vi "Quizz1.vi"() -> ()   [LabVIEW 2020]
uses:
  <vilib>/regexp/Match Regular Expression.xnode
panel:
  out "appended array 2":string[][](array[string])
  out "appended array":string[](array[string])
  out "result string 3":string
  out "result string 2":string
  out "result string":string
  out "LED 3":bool
  in  "PULSADOR 3":bool
  out "LED 2":bool
  in  "PULSADOR 2":bool
  out "LED 1":bool
  in  "PULSADOR 1":bool
  out "Contador":i32
  out "offset past number":i32
  in  "Ingrese la trama":string
  out "Respuestas":string
  in  "Ingreso de comandos":string
  in  "Ingresar":bool
  # "Quiz 1"
  # "Juan Camilo Osorio Bustamante - Diego Alejandro Vallejo Pacheco"
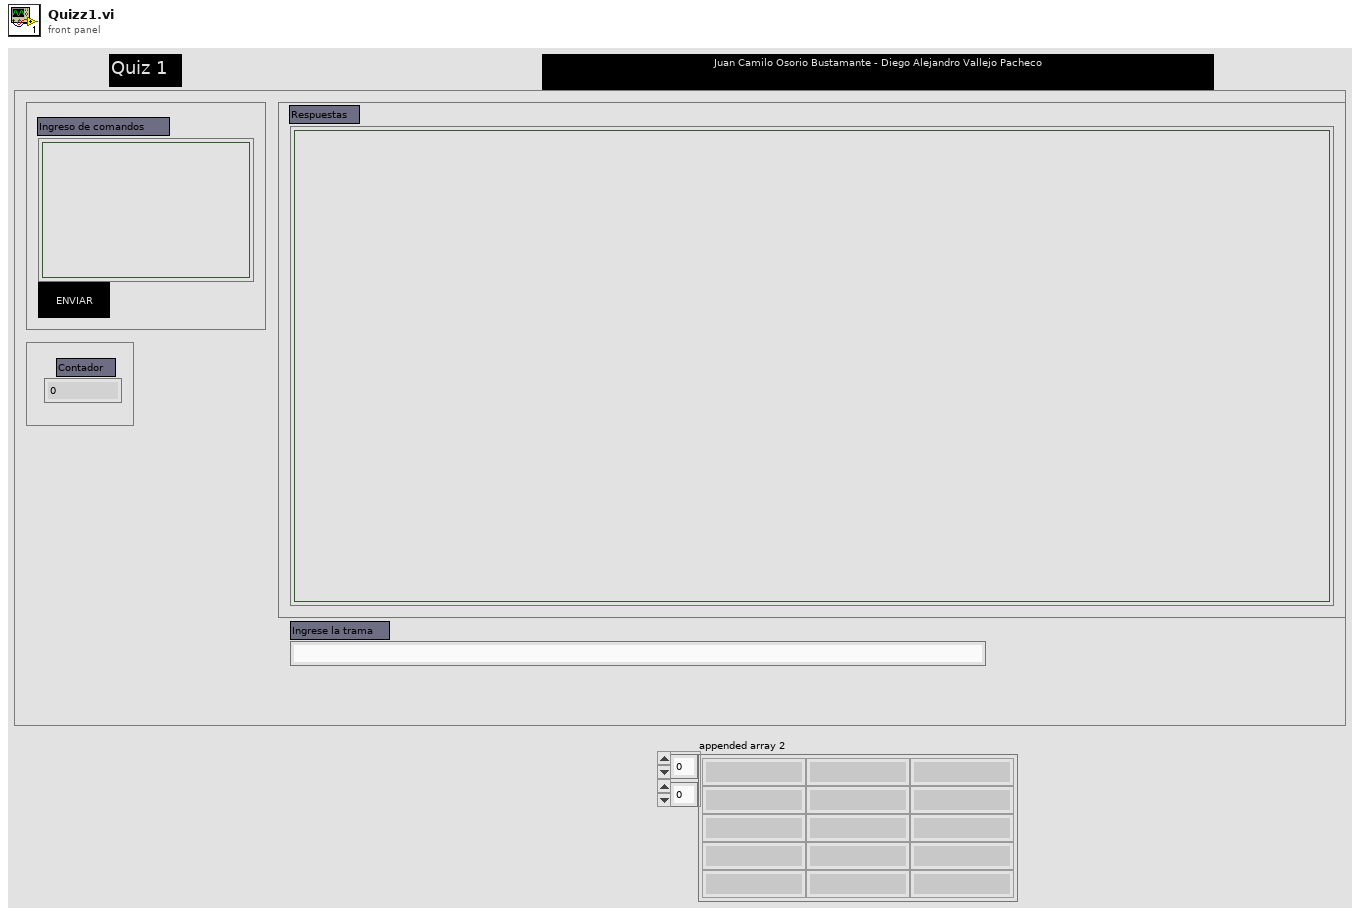
[diagram p1: front panel]
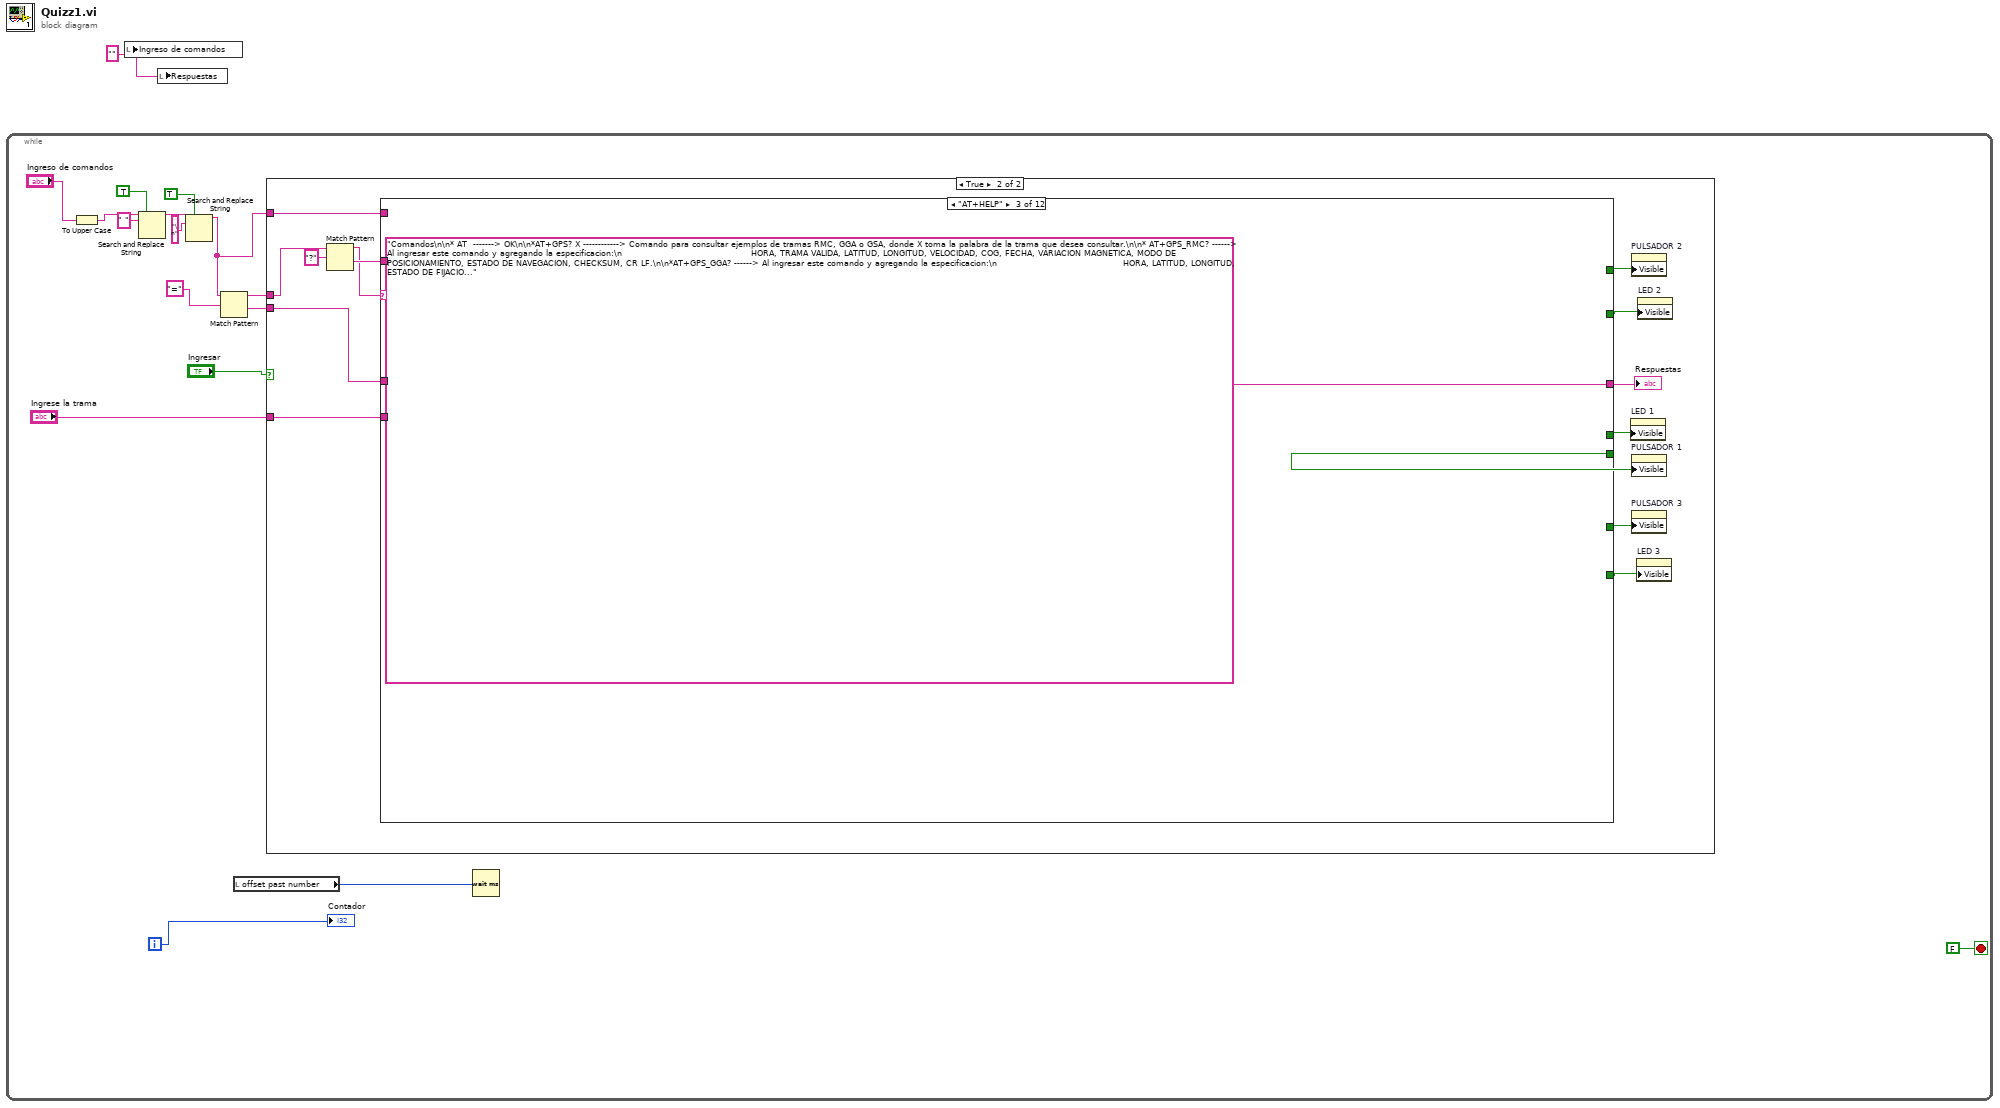
[diagram p0: block diagram]
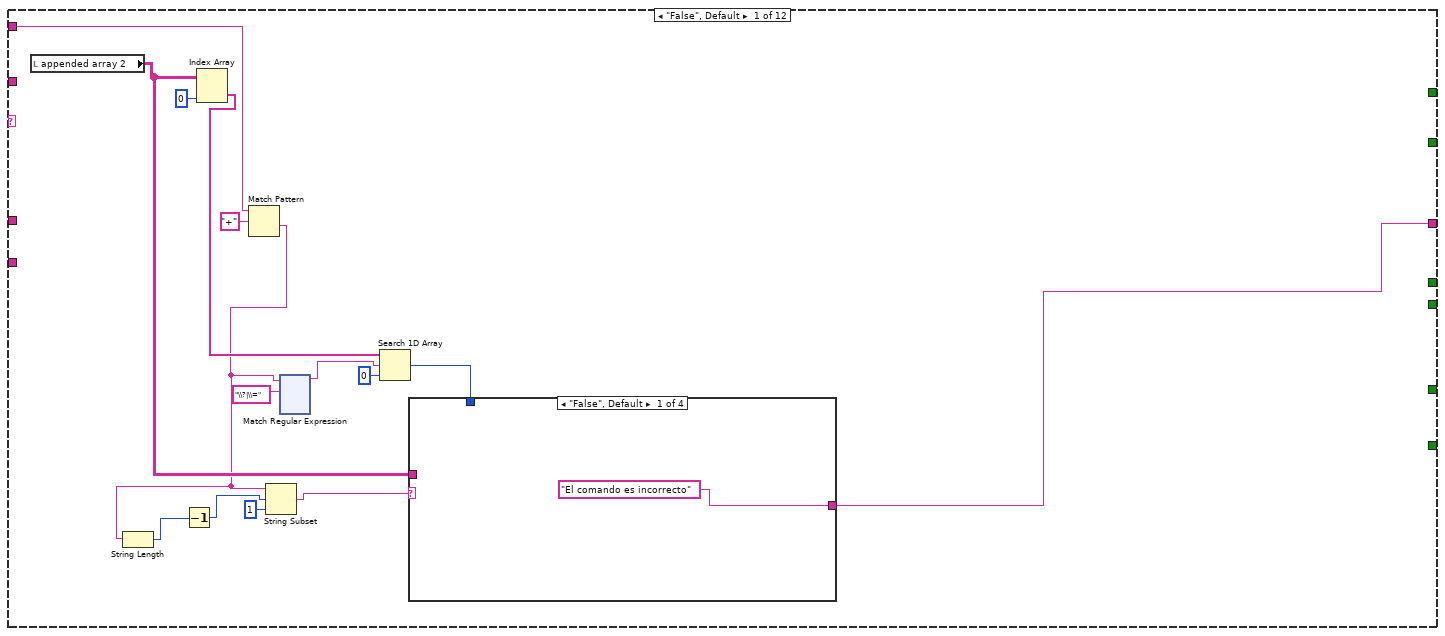
[diagram p3: hidden frame]
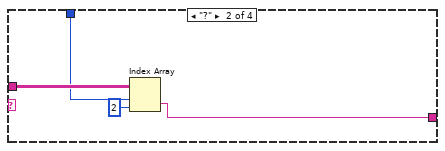
[diagram p4: hidden frame]
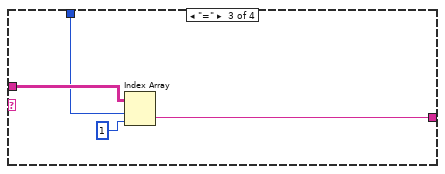
[diagram p5: hidden frame]
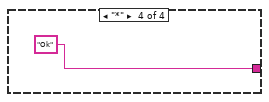
[diagram p6: hidden frame]
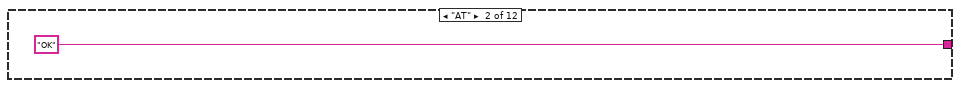
[diagram p7: hidden frame]
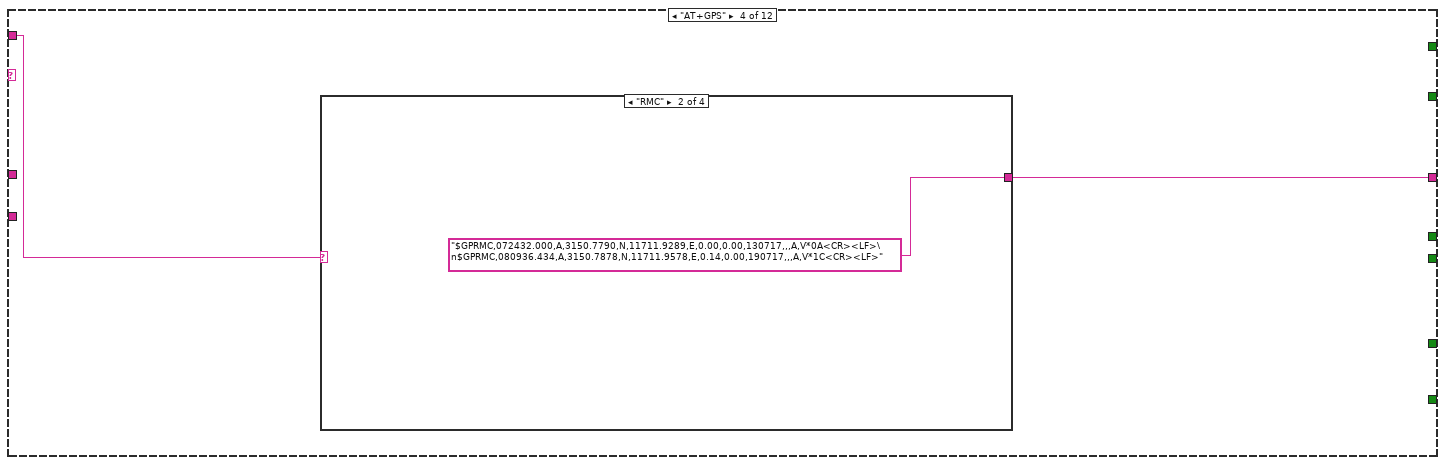
[diagram p8: hidden frame]
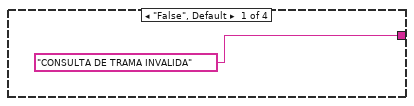
[diagram p9: hidden frame]
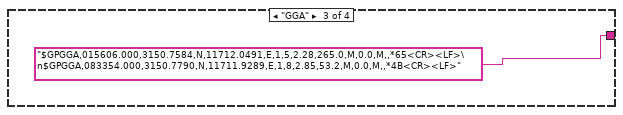
[diagram p10: hidden frame]
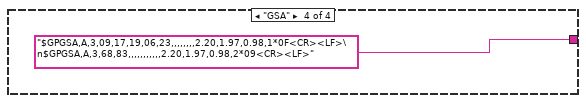
[diagram p11: hidden frame]
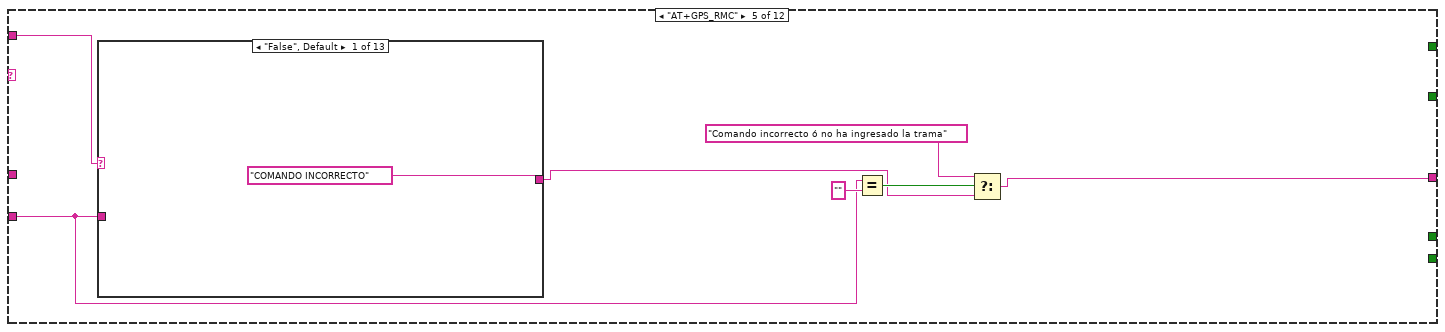
[diagram p12: hidden frame]
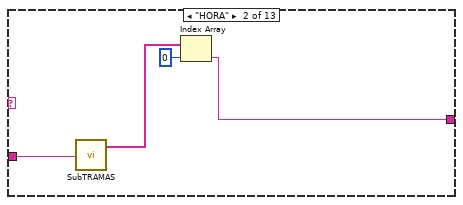
[diagram p13: hidden frame]
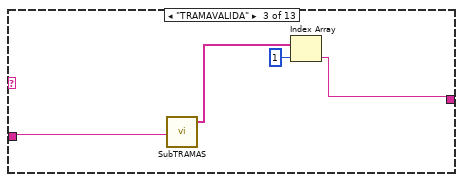
[diagram p14: hidden frame]
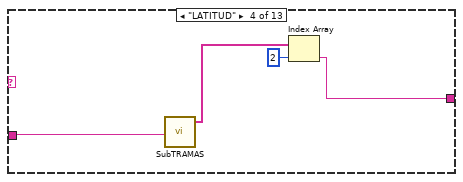
[diagram p15: hidden frame]
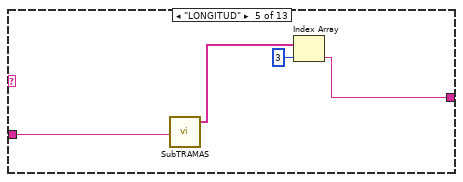
[diagram p16: hidden frame]
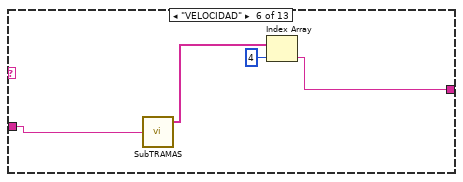
[diagram p17: hidden frame]
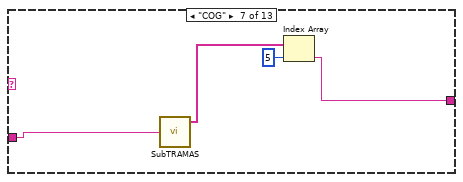
[diagram p18: hidden frame]
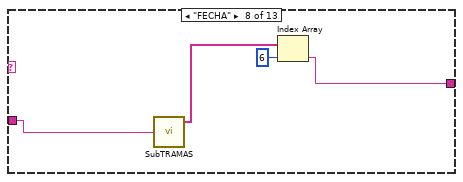
[diagram p19: hidden frame]
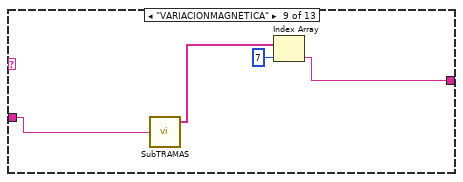
[diagram p20: hidden frame]
diagram:
  w1 = ""
  n1 = while {
    i -> [w4]
    stop <- FALSE stop-if-true
    n2 = To Upper Case(1:"Ingreso de comandos") -> (0:w10:string)
    n3 = Search and Replace String(replace all?=TRUE ("replace all? (F)"), input string=w10, search string=" ") -> (result string=w9:string)  [unwired: 5 in, 3 out]
    n4 = Search and Replace String(replace all?=TRUE ("replace all? (F)"), input string=w9, search string="\n") -> (result string=w3:string)  [unwired: 5 in, 3 out]
    n5 = Match Pattern(string=w3, regular expression="=") -> (before substring=w14:string, after substring=w13:string)  [unwired: 1 in, 2 out]
    n6 = local read "offset past number"() -> (w2:i32)
    n7 = case shown="True" "Ingresar" {
      tunnel: "Ingrese la trama" -> [_ w25]
      tunnel: w14 -> [_ w29]
      tunnel: w13 -> [_ w30]
      tunnel: w3 -> [_ w18]
      frame False {
      }
      frame True {
        n8 = Match Pattern(string=w29, regular expression="?") -> (before substring=w26:string, after substring=w27:string)  [unwired: 1 in, 2 out]
        n9 = case shown="\"AT+HELP\"" w26 {
          tunnel: [w32 "OK" "Comandos\n\n* AT  -------> OK\n\n*AT+GPS? X ------------> Comando para consultar ejemplos de tramas RMC, GGA o GSA, donde X toma la palabra de la trama que desea consultar.\n\n* AT+GPS_RMC? ------> Al ingresar este comando y agregando la especificacion:\n                                           HORA, TRAMA VALIDA, LATITUD, LONGITUD, VELOCIDAD, COG, FECHA, VARIACION MAGNETICA, MODO DE POSICIONAMIENTO, ESTADO DE NAVEGACION, CHECKSUM, CR LF.\n\n*AT+GPS_GGA? ------> Al ingresar este comando y agregando la especificacion:\n                                          HORA, LATITUD, LONGITUD, ESTADO DE FIJACION, NUMERO DE SATELITES EN USO, HDOP, ALTITUD, SEPARACION GEIODE, AÑOS DGPS, ID DE LA ESTACION DGPS, CHECKSUM, CR LF.\n\n*AT+GPS_GSA? ------> Al ingresar este comando y agregando la especificacion:\n                                          MODO, ESTADO DE FIJACION, SATELITES CANAL 1, SATELITES CANAL 2, SATELITES CANAL 3, SATELITES CANAL 4, SATELITES CANAL 5, SATELITES CANAL 6, SATELITES CANAL 7, SATELITES CANAL 8, SATELITES CANAL 9, SATELITES CANAL 10, SATELITES CANAL 11, SATELITES CANAL 12, PDOP, HDOP, VDOP, ID DEL SISTEMA GNSS, CR LF.\n\n*AT+TIEMPO=X --------> Modifica el tiempo en que el contador cambia, donde:\n                                          X es el valor en milisengundos al que desee modificar.\n\n*AT+LEER CONTADOR --> Comando que arroja el tiempo transcurrido del contador en el momento exacto en que se ingresa el comando.\n\n\n*AT+FECHA Y HORA  --> Comando que arroja la hora y fecha actual al momento de ingresar el comando.\n\n*AT+BOTON? X  ------> Comando para modificar el estado de los leds, donde X toma la palabra \"pulsador\", para modificar el estado de estos ó toma la palabra \"leds\", donde se ve el estado de estos.\n\n*AT+INSERTAR? X, Y, Z -----> Comando para insertar un nuevo comando, donde X es el nombre del nuevo comando, Y son las posibles respuestas del comando, Z es la respuesta que quiere del comando. (Ejemplo: AT+Genero*--> Ok, AT+Genero--> posibles respuestas, AT+Genero? --> respuestas)" w173 w179 w235 w291 "Tiempo modificado" w382 w385 w388 "Comando agregado correctamente"] -> w31
          tunnel: w25 -> [_ _ _ _ w182 w237 w292 _ _ _ _ _]
          tunnel: w30 -> [_ _ _ _ _ _ _ w380 _ _ _ _]
          tunnel: w27 -> [_ _ _ w174 w185 w241 w297 _ _ _ w389 w407]
          tunnel: [_ _ _ _ _ _ _ _ _ _ w386 _] -> w24
          tunnel: [_ _ _ _ _ _ _ _ _ _ w387 _] -> w23
          tunnel: [_ _ _ _ _ _ _ _ _ _ w386 _] -> w22
          tunnel: [_ _ _ _ _ _ _ _ _ _ w387 _] -> w21
          tunnel: [_ _ _ _ _ _ _ _ _ _ w387 _] -> w20
          tunnel: [_ _ _ _ _ _ _ _ _ _ w386 _] -> w19
          tunnel: w18 -> [w43 _ _ _ _ _ _ _ _ _ _ _]
          frame "False", Default {
            n10 = local read "appended array 2"() -> (w39:string[][])
            n11 = Index Array(array=w39, index (col)=0 ("disabled index (col)")) -> (element=w42:string[])  [unwired: 1 in]
            n12 = Match Pattern(string=w43, regular expression="+") -> (after substring=w34:string)  [unwired: 1 in, 3 out]
            n13 = String Length(string=w34) -> (length=w38:i32)
            n14 = Decrement(x=w38) -> (x-1=w37:i32)
            n15 = String Subset(string=w34, offset (0)=w37, length (rest)=1 ("length (rest)")) -> (substring=w40:string)
            n16 = xnode "Match Regular Expression"("input string"=w34, "regular expression"="\\?|\\=") -> ("before match"=w35:string)  [unwired: 4 in, 4 out]
            n17 = Search 1D Array(1D array=w42, element=w35, start index (0)=0) -> (index of element=w33:i32)
            n18 = case shown="\"False\", Default" w40 {
              tunnel: w39 -> [_ w165 w169 _]
              tunnel: w33 -> [_ w164 w168 _]
              tunnel: ["El comando es incorrecto" w162 w166 "Ok"] -> w32
              frame "False", Default {
              }
              frame "?" {
                n19 = Index Array(array=w165, index (row)=w164, index (col)=2 ("disabled index (col)")) -> (element=w162:string)
              }
              frame "=" {
                n20 = Index Array(array=w169, index (row)=w168, index (col)=1 ("disabled index (col)")) -> (element=w166:string)
              }
              frame "*" {
              }
            }
          }
          frame "AT" {
          }
          frame "AT+HELP" {
          }
          frame "AT+GPS" {
            n21 = case shown="\"RMC\"" w174 {
              tunnel: ["CONSULTA DE TRAMA INVALIDA" "$GPRMC,072432.000,A,3150.7790,N,11711.9289,E,0.00,0.00,130717,,,A,V*0A<CR><LF>\n$GPRMC,080936.434,A,3150.7878,N,11711.9578,E,0.14,0.00,190717,,,A,V*1C<CR><LF>" "$GPGGA,015606.000,3150.7584,N,11712.0491,E,1,5,2.28,265.0,M,0.0,M,,*65<CR><LF>\n$GPGGA,083354.000,3150.7790,N,11711.9289,E,1,8,2.85,53.2,M,0.0,M,,*4B<CR><LF>" "$GPGSA,A,3,09,17,19,06,23,,,,,,,,2.20,1.97,0.98,1*0F<CR><LF>\n$GPGSA,A,3,68,83,,,,,,,,,,,2.20,1.97,0.98,2*09<CR><LF>"] -> w173
              frame "False", Default {
              }
              frame "RMC" {
              }
              frame "GGA" {
              }
              frame "GSA" {
              }
            }
          }
          frame "AT+GPS_RMC" {
            n22 = case shown="\"False\", Default" w185 {
              tunnel: ["COMANDO INCORRECTO" w187 w191 w196 w200 w203 w207 w211 w215 w219 w223 w227 w231] -> w181
              tunnel: w182 -> [_ w188 w192 w195 w199 w204 w208 w212 w216 w220 w224 w228 w232]
              frame "False", Default {
              }
              frame "HORA" {
                n23 = call "SubTRAMAS.vi"("Trama"=w188) -> ("RMC"=w190:string[])  [unwired: 2 out]
                n24 = Index Array(array=w190, index=0) -> (element=w187:string)
              }
              frame "TRAMAVALIDA" {
                n25 = call "SubTRAMAS.vi"("Trama"=w192) -> ("RMC"=w194:string[])  [unwired: 2 out]
                n26 = Index Array(array=w194, index=1) -> (element=w191:string)
              }
              frame "LATITUD" {
                n27 = call "SubTRAMAS.vi"("Trama"=w195) -> ("RMC"=w198:string[])  [unwired: 2 out]
                n28 = Index Array(array=w198, index=2) -> (element=w196:string)
              }
              frame "LONGITUD" {
                n29 = call "SubTRAMAS.vi"("Trama"=w199) -> ("RMC"=w202:string[])  [unwired: 2 out]
                n30 = Index Array(array=w202, index=3) -> (element=w200:string)
              }
              frame "VELOCIDAD" {
                n31 = call "SubTRAMAS.vi"("Trama"=w204) -> ("RMC"=w206:string[])  [unwired: 2 out]
                n32 = Index Array(array=w206, index=4) -> (element=w203:string)
              }
              frame "COG" {
                n33 = call "SubTRAMAS.vi"("Trama"=w208) -> ("RMC"=w210:string[])  [unwired: 2 out]
                n34 = Index Array(array=w210, index=5) -> (element=w207:string)
              }
              frame "FECHA" {
                n35 = call "SubTRAMAS.vi"("Trama"=w212) -> ("RMC"=w214:string[])  [unwired: 2 out]
                n36 = Index Array(array=w214, index=6) -> (element=w211:string)
              }
              frame "VARIACIONMAGNETICA" {
                n37 = call "SubTRAMAS.vi"("Trama"=w216) -> ("RMC"=w218:string[])  [unwired: 2 out]
                n38 = Index Array(array=w218, index=7) -> (element=w215:string)
              }
              frame "MODODEPOSICIONAMIENTO" {
                n39 = call "SubTRAMAS.vi"("Trama"=w220) -> ("RMC"=w222:string[])  [unwired: 2 out]
                n40 = Index Array(array=w222, index=8) -> (element=w219:string)
              }
              frame "ESTADODENAVEGACION" {
                n41 = call "SubTRAMAS.vi"("Trama"=w224) -> ("RMC"=w226:string[])  [unwired: 2 out]
                n42 = Index Array(array=w226, index=9) -> (element=w223:string)
              }
              frame "CHECKSUM" {
                n43 = call "SubTRAMAS.vi"("Trama"=w228) -> ("RMC"=w230:string[])  [unwired: 2 out]
                n44 = Index Array(array=w230, index=10) -> (element=w227:string)
              }
              frame "CRLF" {
                n45 = call "SubTRAMAS.vi"("Trama"=w232) -> ("RMC"=w234:string[])  [unwired: 2 out]
                n46 = Index Array(array=w234, index=11) -> (element=w231:string)
              }
            }
            n47 = Equal?(x=w182, y="") -> (x = y?=w183:bool)
            n48 = Select(t="Comando incorrecto ó no ha ingresado la trama", s=w183, f=w181) -> (s? t:f=w179:string)
          }
          frame "AT+GPS_GGA" {
            n49 = case shown="\"False\", Default" w241 {
              tunnel: w237 -> [_ w245 w248 w252 w256 w260 w264 w268 w272 w276 w280 w284 w288]
              tunnel: ["COMANDO INCORRECTO" w243 w247 w251 w255 w259 w263 w267 w271 w275 w279 w283 w287] -> w236
              frame "False", Default {
              }
              frame "HORA" {
                n50 = call "SubTRAMAS.vi"("Trama"=w245) -> ("GGA"=w244:string[])  [unwired: 2 out]
                n51 = Index Array(array=w244, index=0) -> (element=w243:string)
              }
              frame "LATITUD" {
                n52 = call "SubTRAMAS.vi"("Trama"=w248) -> ("GGA"=w249:string[])  [unwired: 2 out]
                n53 = Index Array(array=w249, index=1) -> (element=w247:string)
              }
              frame "LONGITUD" {
                n54 = call "SubTRAMAS.vi"("Trama"=w252) -> ("GGA"=w253:string[])  [unwired: 2 out]
                n55 = Index Array(array=w253, index=2) -> (element=w251:string)
              }
              frame "ESTADODEFIJACION" {
                n56 = call "SubTRAMAS.vi"("Trama"=w256) -> ("GGA"=w257:string[])  [unwired: 2 out]
                n57 = Index Array(array=w257, index=3) -> (element=w255:string)
              }
              frame "NUMERODESATELITESENUSO" {
                n58 = call "SubTRAMAS.vi"("Trama"=w260) -> ("GGA"=w261:string[])  [unwired: 2 out]
                n59 = Index Array(array=w261, index=4) -> (element=w259:string)
              }
              frame "HDOP" {
                n60 = call "SubTRAMAS.vi"("Trama"=w264) -> ("GGA"=w265:string[])  [unwired: 2 out]
                n61 = Index Array(array=w265, index=5) -> (element=w263:string)
              }
              frame "ALTITUD" {
                n62 = call "SubTRAMAS.vi"("Trama"=w268) -> ("GGA"=w269:string[])  [unwired: 2 out]
                n63 = Index Array(array=w269, index=6) -> (element=w267:string)
              }
              frame "SEPARACIONGEOIDE" {
                n64 = call "SubTRAMAS.vi"("Trama"=w272) -> ("GGA"=w273:string[])  [unwired: 2 out]
                n65 = Index Array(array=w273, index=7) -> (element=w271:string)
              }
              frame "AÑOSDGPS" {
                n66 = call "SubTRAMAS.vi"("Trama"=w276) -> ("GGA"=w277:string[])  [unwired: 2 out]
                n67 = Index Array(array=w277, index=8) -> (element=w275:string)
              }
              frame "IDDELAESTACIONDGPS" {
                n68 = call "SubTRAMAS.vi"("Trama"=w280) -> ("GGA"=w281:string[])  [unwired: 2 out]
                n69 = Index Array(array=w281, index=9) -> (element=w279:string)
              }
              frame "CHECKSUM" {
                n70 = call "SubTRAMAS.vi"("Trama"=w284) -> ("GGA"=w285:string[])  [unwired: 2 out]
                n71 = Index Array(array=w285, index=10) -> (element=w283:string)
              }
              frame "CRLF" {
                n72 = call "SubTRAMAS.vi"("Trama"=w288) -> ("GGA"=w289:string[])  [unwired: 2 out]
                n73 = Index Array(array=w289, index=11) -> (element=w287:string)
              }
            }
            n74 = Equal?(x=w237, y="") -> (x = y?=w239:bool)
            n75 = Select(t="Comando incorrecto ó no ha ingresado la trama", s=w239, f=w236) -> (s? t:f=w235:string)
          }
          frame "AT+GPS_GSA" {
            n76 = case shown="\"False\", Default" w297 {
              tunnel: w292 -> [_ w301 w304 w308 w312 w316 w320 w324 w328 w333 w336 w340 w344 w348 w352 w356 w360 w364 w368 w372 w376]
              tunnel: ["COMANDO INCORRECTO" w299 w303 w307 w311 w315 w319 w323 w327 w332 w335 w339 w343 w347 w351 w355 w359 w363 w367 w371 w375] -> w293
              frame "False", Default {
              }
              frame "MODO" {
                n77 = call "SubTRAMAS.vi"("Trama"=w301) -> ("GSA"=w300:string[])  [unwired: 2 out]
                n78 = Index Array(array=w300, index=0) -> (element=w299:string)
              }
              frame "ESTADODEFIJACION" {
                n79 = call "SubTRAMAS.vi"("Trama"=w304) -> ("GSA"=w305:string[])  [unwired: 2 out]
                n80 = Index Array(array=w305, index=1) -> (element=w303:string)
              }
              frame "SATELITESCANAL1" {
                n81 = call "SubTRAMAS.vi"("Trama"=w308) -> ("GSA"=w309:string[])  [unwired: 2 out]
                n82 = Index Array(array=w309, index=2) -> (element=w307:string)
              }
              frame "SATELITESCANAL2" {
                n83 = call "SubTRAMAS.vi"("Trama"=w312) -> ("GSA"=w313:string[])  [unwired: 2 out]
                n84 = Index Array(array=w313, index=3) -> (element=w311:string)
              }
              frame "SATELITESCANAL3" {
                n85 = call "SubTRAMAS.vi"("Trama"=w316) -> ("GSA"=w317:string[])  [unwired: 2 out]
                n86 = Index Array(array=w317, index=4) -> (element=w315:string)
              }
              frame "SATELITESCANAL4" {
                n87 = call "SubTRAMAS.vi"("Trama"=w320) -> ("GSA"=w321:string[])  [unwired: 2 out]
                n88 = Index Array(array=w321, index=5) -> (element=w319:string)
              }
              frame "SATELITESCANAL5" {
                n89 = call "SubTRAMAS.vi"("Trama"=w324) -> ("GSA"=w325:string[])  [unwired: 2 out]
                n90 = Index Array(array=w325, index=6) -> (element=w323:string)
              }
              frame "SATELITESCANAL6" {
                n91 = call "SubTRAMAS.vi"("Trama"=w328) -> ("GSA"=w329:string[])  [unwired: 2 out]
                n92 = Index Array(array=w329, index=7) -> (element=w327:string)
              }
              frame "SATELITESCANAL7" {
                n93 = call "SubTRAMAS.vi"("Trama"=w333) -> ("GSA"=w334:string[])  [unwired: 2 out]
                n94 = Index Array(array=w334, index=8) -> (element=w332:string)
              }
              frame "SATELITESCANAL8" {
                n95 = call "SubTRAMAS.vi"("Trama"=w336) -> ("GSA"=w337:string[])  [unwired: 2 out]
                n96 = Index Array(array=w337, index=9) -> (element=w335:string)
              }
              frame "SATELITESCANAL9" {
                n97 = call "SubTRAMAS.vi"("Trama"=w340) -> ("GSA"=w341:string[])  [unwired: 2 out]
                n98 = Index Array(array=w341, index=10) -> (element=w339:string)
              }
              frame "SATELITESCANAL10" {
                n99 = call "SubTRAMAS.vi"("Trama"=w344) -> ("GSA"=w345:string[])  [unwired: 2 out]
                n100 = Index Array(array=w345, index=11) -> (element=w343:string)
              }
              frame "SATELITESCANAL11" {
                n101 = call "SubTRAMAS.vi"("Trama"=w348) -> ("GSA"=w349:string[])  [unwired: 2 out]
                n102 = Index Array(array=w349, index=12) -> (element=w347:string)
              }
              frame "SATELITESCANAL12" {
                n103 = call "SubTRAMAS.vi"("Trama"=w352) -> ("GSA"=w353:string[])  [unwired: 2 out]
                n104 = Index Array(array=w353, index=13) -> (element=w351:string)
              }
              frame "PDOP" {
                n105 = call "SubTRAMAS.vi"("Trama"=w356) -> ("GSA"=w357:string[])  [unwired: 2 out]
                n106 = Index Array(array=w357, index=14) -> (element=w355:string)
              }
              frame "HDOP" {
                n107 = call "SubTRAMAS.vi"("Trama"=w360) -> ("GSA"=w361:string[])  [unwired: 2 out]
                n108 = Index Array(array=w361, index=15) -> (element=w359:string)
              }
              frame "VDOP" {
                n109 = call "SubTRAMAS.vi"("Trama"=w364) -> ("GSA"=w365:string[])  [unwired: 2 out]
                n110 = Index Array(array=w365, index=16) -> (element=w363:string)
              }
              frame "IDDELSISTEMAGNSS" {
                n111 = call "SubTRAMAS.vi"("Trama"=w368) -> ("GSA"=w369:string[])  [unwired: 2 out]
                n112 = Index Array(array=w369, index=17) -> (element=w367:string)
              }
              frame "CHECKSUM" {
                n113 = call "SubTRAMAS.vi"("Trama"=w372) -> ("GSA"=w374:string[])  [unwired: 2 out]
                n114 = Index Array(array=w374, index=18) -> (element=w371:string)
              }
              frame "CRLF" {
                n115 = call "SubTRAMAS.vi"("Trama"=w376) -> ("GSA"=w378:string[])  [unwired: 2 out]
                n116 = Index Array(array=w378, index=19) -> (element=w375:string)
              }
            }
            n117 = Equal?(x=w292, y="") -> (x = y?=w295:bool)
            n118 = Select(t="Comando incorrecto ó no ha ingresado la trama", s=w295, f=w293) -> (s? t:f=w291:string)
          }
          frame "AT+TIEMPO" {
            n119 = Decimal String To Number(string=w380) -> (number=→"offset past number":i32)  [unwired: 2 in, 1 out]
          }
          frame "AT+LEERCONTADOR" {
            n120 = local read "Contador"() -> (w383:i32)
            n121 = Number To Decimal String(number=w383) -> (decimal integer string=w382:string)  [unwired: 1 in]
          }
          frame "AT+FECHAYHORA" {
            n122 = Format Date/Time String(time format string (%c)="Hora:\n%H:%M:%S\n\nFecha:\n%d/%m/%y" ("regular expression")) -> (date/time string=w385:string)  [unwired: 2 in]
          }
          frame "AT+BOTON" {
            n123 = case shown="\"LEDS\"" w389 {
              selector: w389 -> [_ w396 w401]
              tunnel: [_ w394 _] -> w386
              tunnel: [_ _ w400] -> w387
              tunnel: ["El comando ingresado no es valido" _ _] -> w388
              frame "False", Default {
              }
              frame "PULSADOR" {
                n124 = Equal?(x=w396, y="PULSADOR") -> (x = y?=w394:bool)
                "LED 1" <- "PULSADOR 1"
                "LED 2" <- "PULSADOR 2"
                "LED 3" <- "PULSADOR 3"
              }
              frame "LEDS" {
                n125 = Equal?(x=w401, y="LEDS") -> (x = y?=w400:bool)
                n126 = local read "PULSADOR 3"() -> (w397:bool)
                n127 = local read "PULSADOR 2"() -> (w398:bool)
                n128 = local read "PULSADOR 1"() -> (w399:bool)
                n129 = local write "LED 1"(w399) -> ()
                n130 = local write "LED 3"(w397) -> ()
                n131 = local write "LED 2"(w398) -> ()
              }
            }
          }
          frame "AT+INSERTAR" {
            n132 = Search and Replace String(replace all?=TRUE ("replace all? (F)"), input string=w407, search string=",", replace string="," ("replace string (\"\")")) -> (number of replacements=w410:i32)  [unwired: 4 in, 3 out]
            n133 = Add(x=w410, y=1) -> (x+y=w408:i32)
            n134 = for {
              N: w408 -> [_]
              shift-right: [w419] -> _
              shift-left: w407 -> [w423]
              tunnel: [w414] -> w406
              i -> [w421]
              n135 = Match Pattern(string=w423, regular expression=",") -> (before substring=w420:string, after substring=w419:string)  [unwired: 1 in, 2 out]
              n136 = Wait (ms)(milliseconds to wait=u32 100) -> ()  [unwired: 1 out]
              n137 = case shown="0" w421 {
                tunnel: w420 -> [_ w424 w425 w426]
                frame 99, Default {
                }
                frame 0 {
                  "result string" <- w424
                }
                frame 1 {
                  "result string 2" <- w425
                }
                frame 2 {
                  "result string 3" <- w426
                }
              }
              n138 = local read "result string 3"() -> (w415:string)
              n139 = local read "result string 2"() -> (w416:string)
              n140 = local read "result string"() -> (w417:string)
              n141 = Build Array(w417, w416, w415) -> (w414:string[])
              "appended array" <- w414
            }
            n142 = local read "appended array 2"() -> (w404:string[][])
            n143 = Build Array (concatenate)(w404, w406) -> (→"appended array 2":string[][])
          }
        }
        "Respuestas" <- w31
        n144 = property on="LED 1" class="Bool (strict)"("Visible"=w23) -> ()  [unwired: 2 in, 2 out]
        n145 = property on="PULSADOR 2" class="Bool (strict)"("Visible"=w22) -> ()  [unwired: 2 in, 2 out]
        n146 = property on="PULSADOR 1" class="Bool (strict)"("Visible"=w24) -> ()  [unwired: 2 in, 2 out]
        n147 = property on="PULSADOR 3" class="Bool (strict)"("Visible"=w19) -> ()  [unwired: 2 in, 2 out]
        n148 = property on="LED 3" class="Bool (strict)"("Visible"=w20) -> ()  [unwired: 2 in, 2 out]
        n149 = property on="LED 2" class="Bool (strict)"("Visible"=w21) -> ()  [unwired: 2 in, 2 out]
      }
    }
    n150 = Wait (ms)(milliseconds to wait=w2) -> ()  [unwired: 1 out]
    "Contador" <- w4
  }
  n151 = local write "Ingreso de comandos"(w1) -> ()
  n152 = local write "Respuestas"(w1) -> ()
